vi "main.vi"() -> ()   [LabVIEW 2019]
uses:
  Controls/data.ctl
  Estats.ctl
panel:
  out "Pict Ring":u16(ring)
  in  "Prova":bool
  out "Diners":string
  in  "Stop Button":bool
  out "Diàleg":string
  out "Canvi":string
  in  "Orange":bool
  in  "Lemond":bool
  in  "Apple":bool
  in  "50cents":bool
  in  "20cents":bool
  in  "10cents":bool
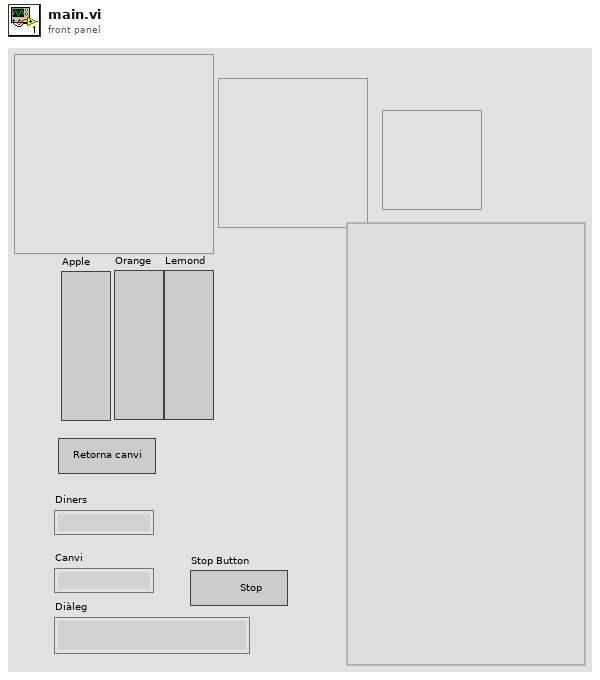
[diagram p1: front panel]
types:
  T1 = typedef "Estats.ctl" = enum16{"Init", "Wait for Event", "Exit", "Return Money", "Lemond", "Apple", "Orange", "Deliver", "50cents", "20cents", "10cents"}
  T2 = typedef "data.ctl" = cluster{"Diners":dbl, "Han triat veguda":bool}
  T3 = enum8{"Enabled", "Disabled", "Disabled and Grayed Out"}
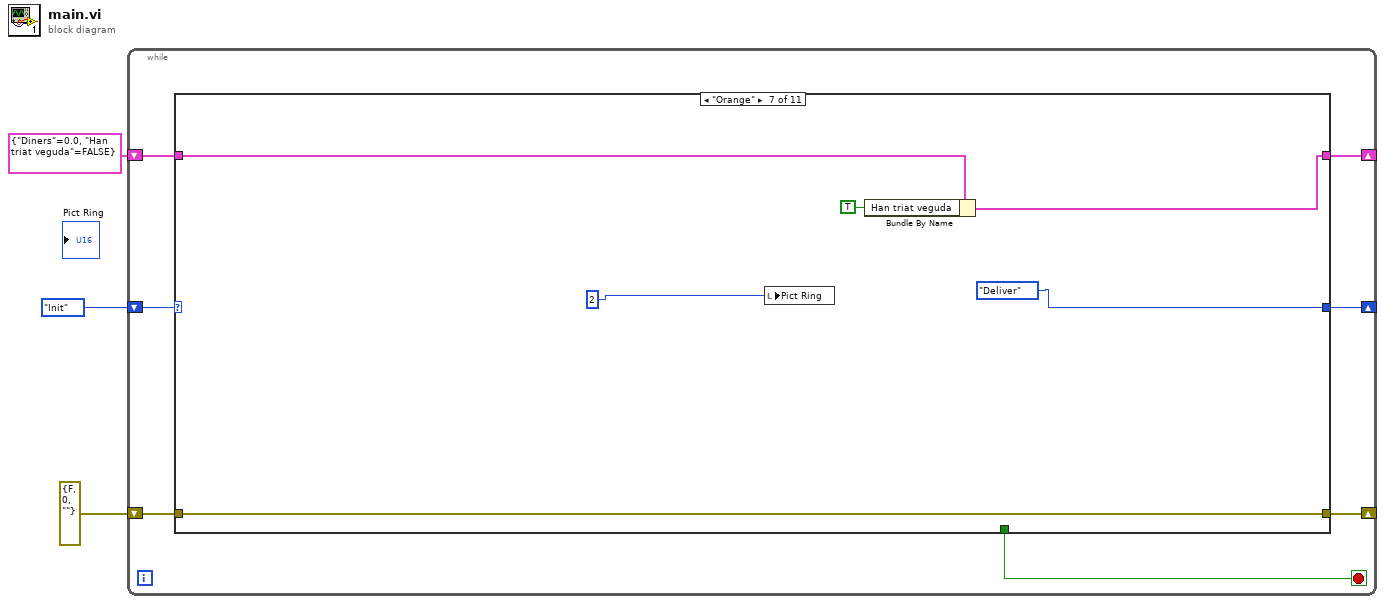
[diagram p0: block diagram]
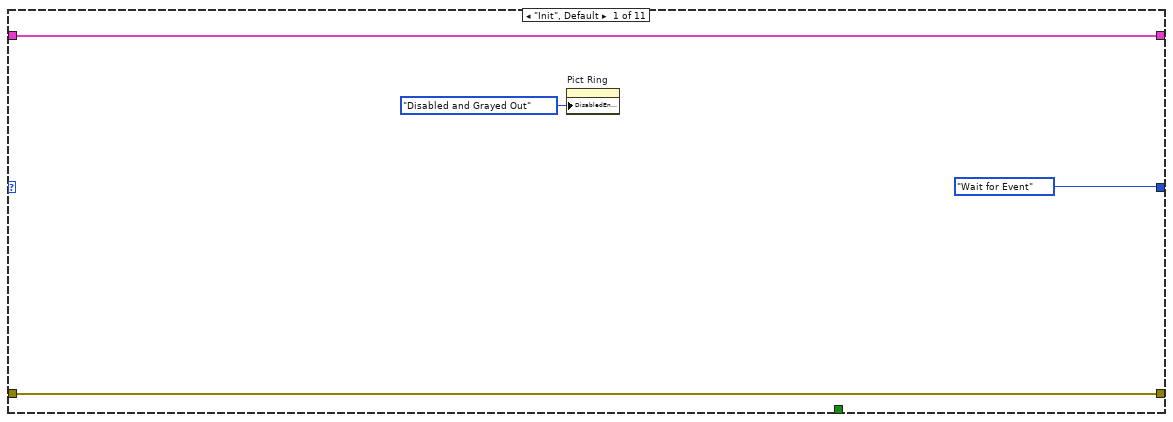
[diagram p2: hidden frame]
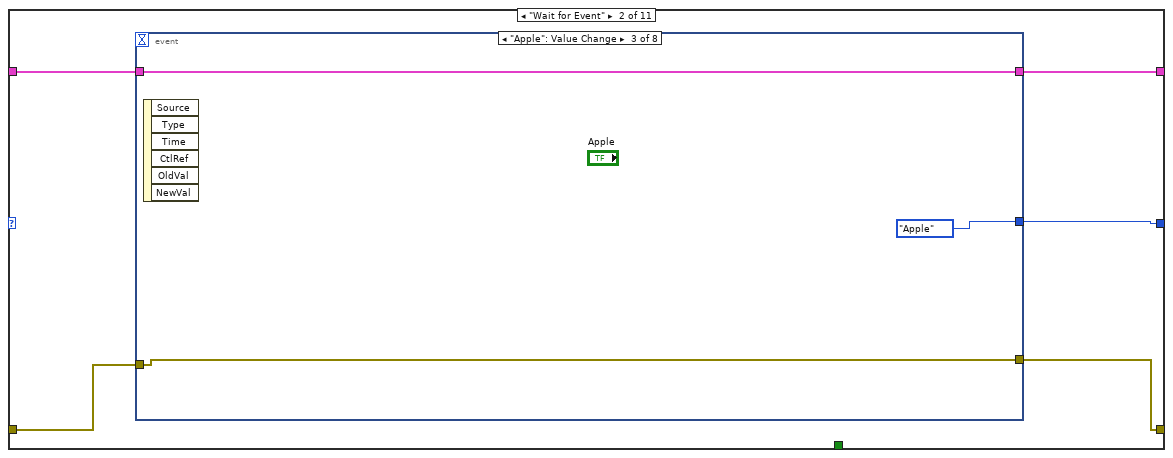
[diagram p3: hidden frame]
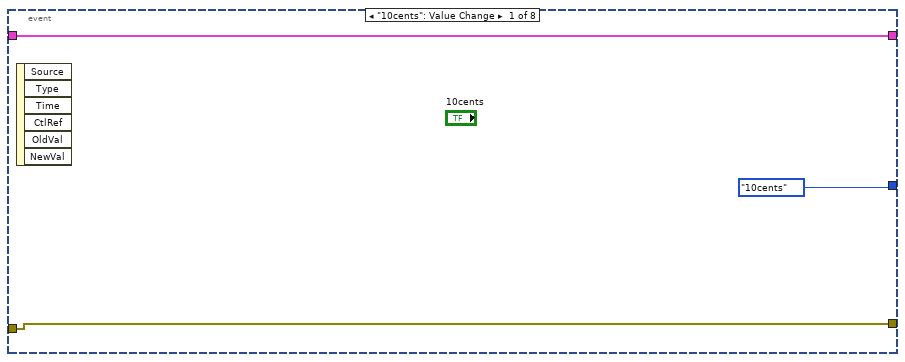
[diagram p4: hidden frame]
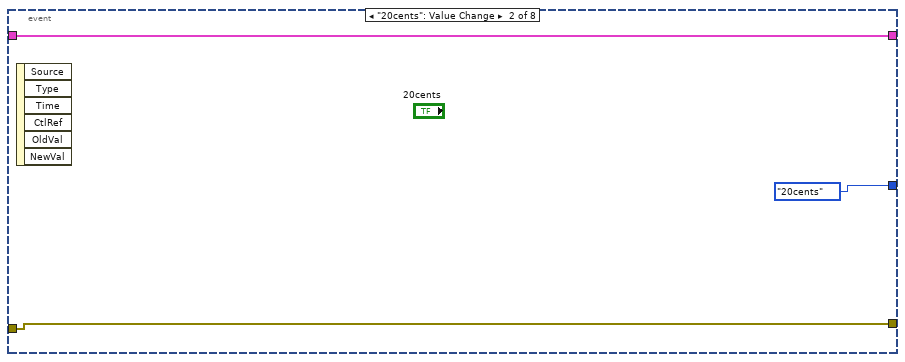
[diagram p5: hidden frame]
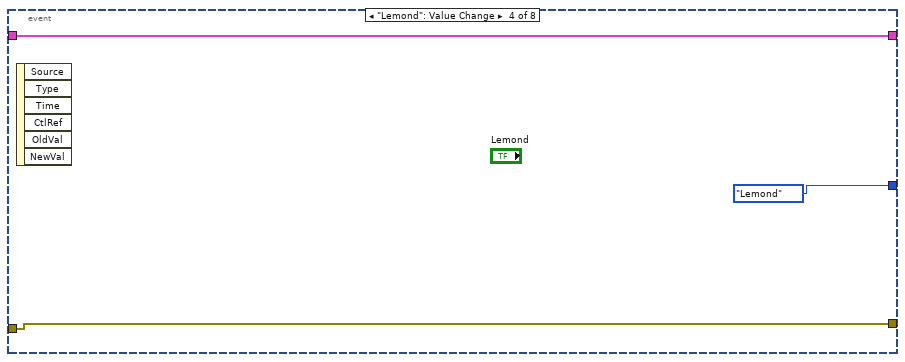
[diagram p6: hidden frame]
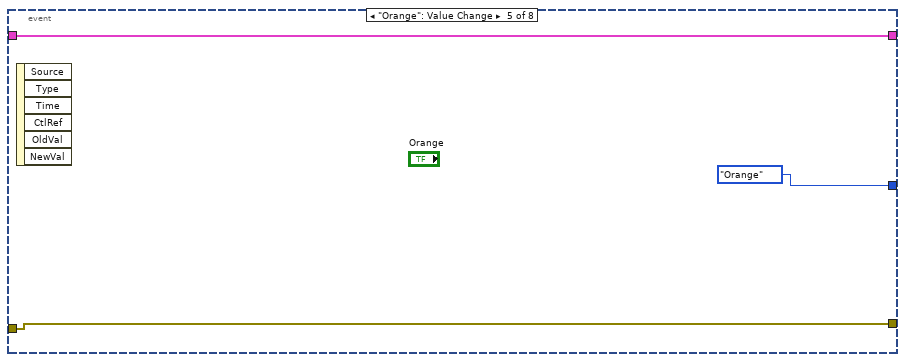
[diagram p7: hidden frame]
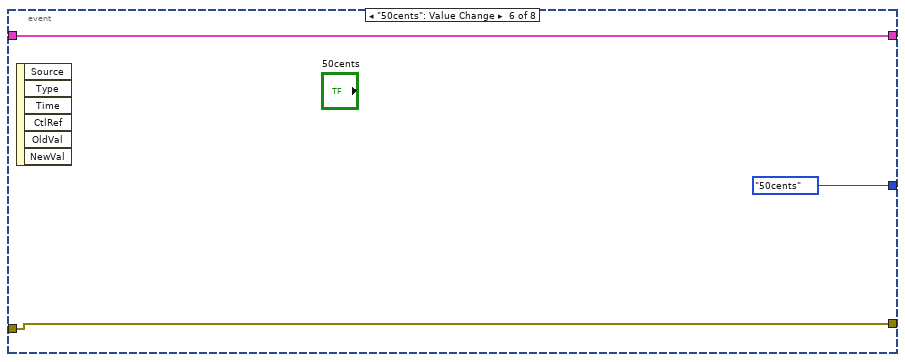
[diagram p8: hidden frame]
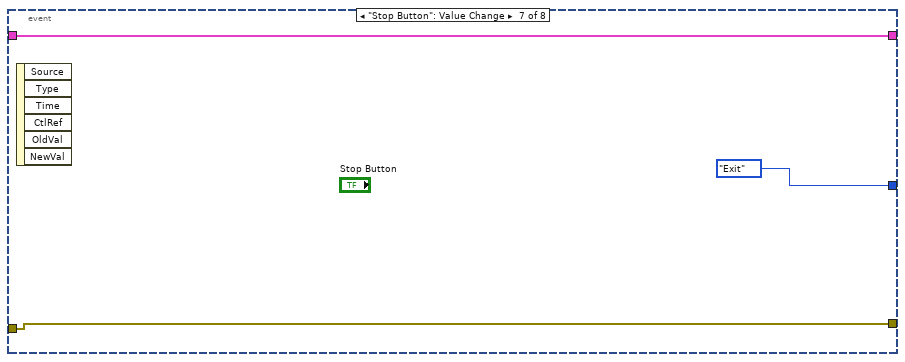
[diagram p9: hidden frame]
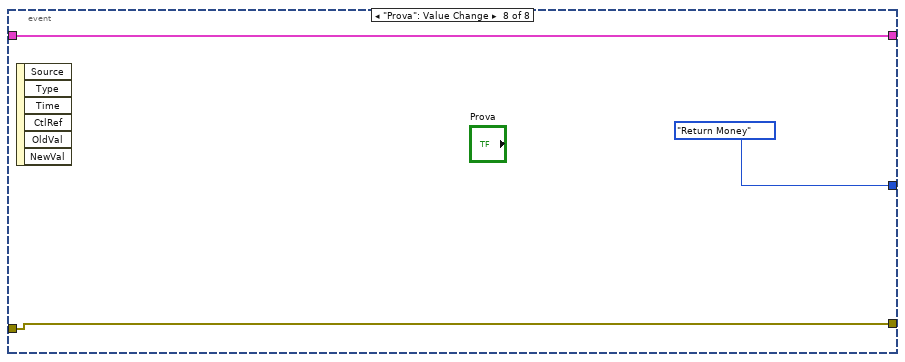
[diagram p10: hidden frame]
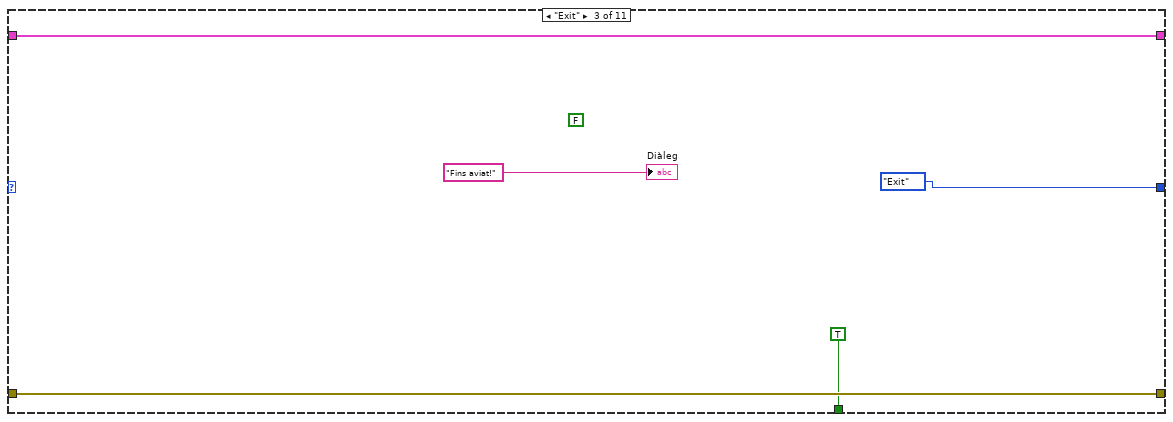
[diagram p11: hidden frame]
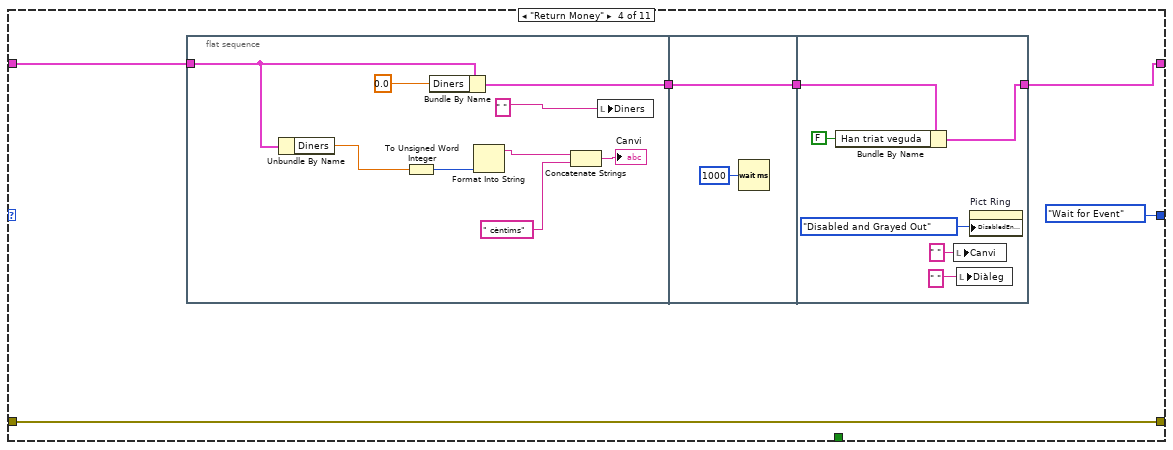
[diagram p12: hidden frame]
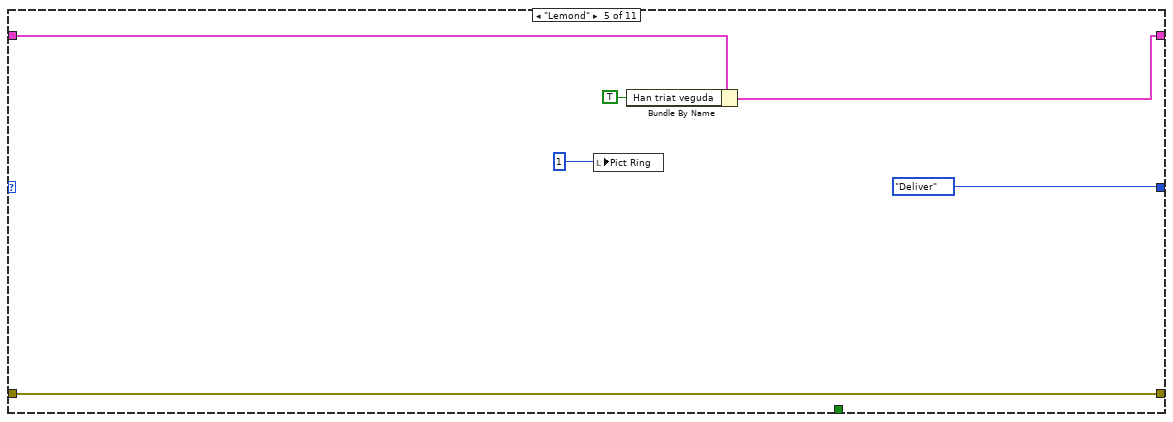
[diagram p13: hidden frame]
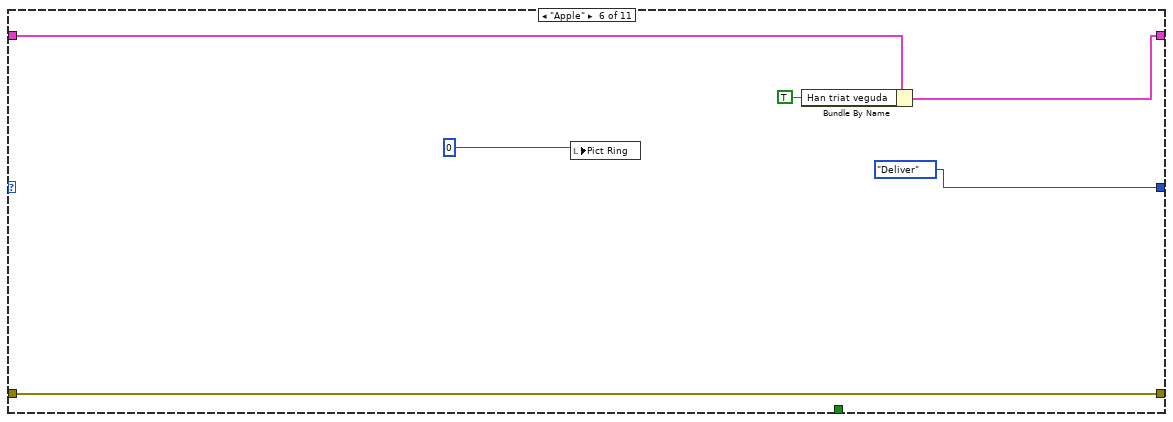
[diagram p14: hidden frame]
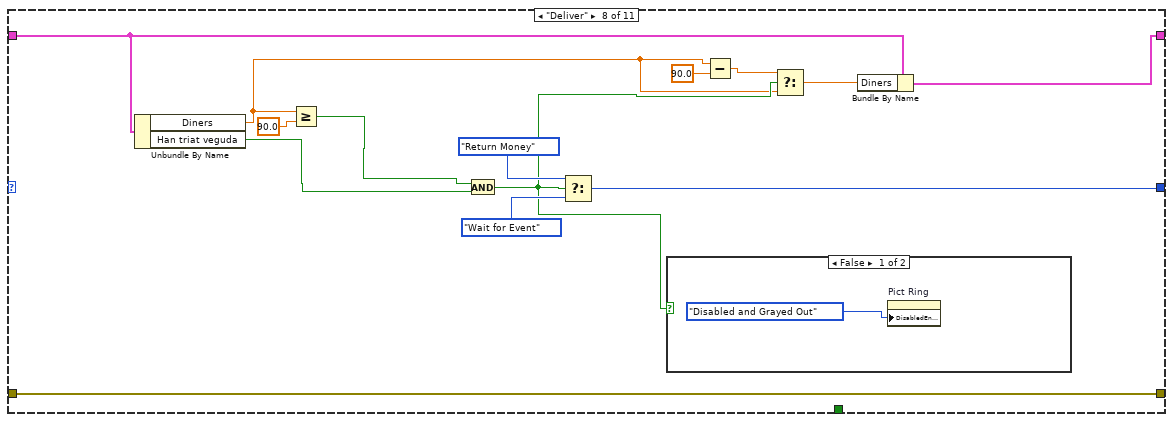
[diagram p15: hidden frame]
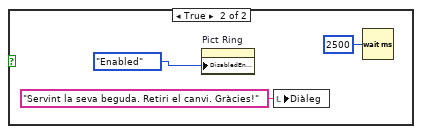
[diagram p16: hidden frame]
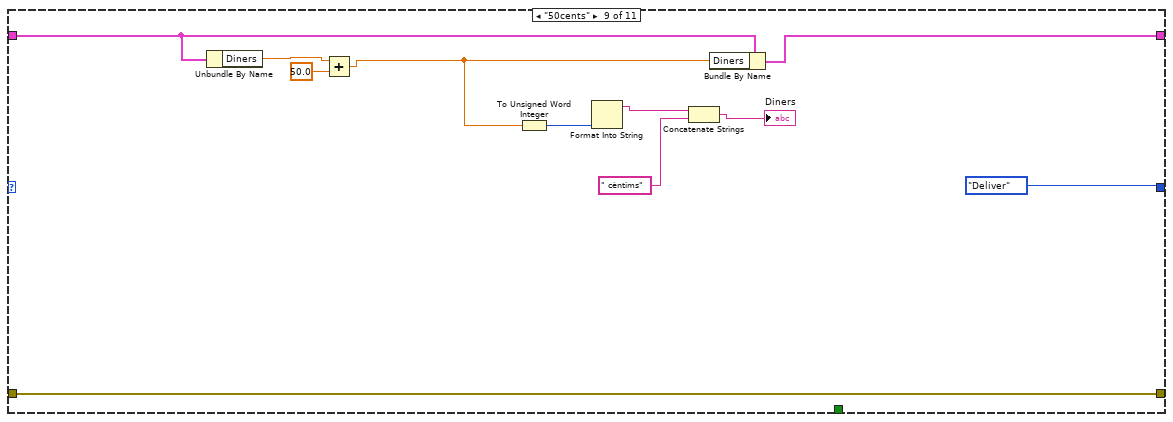
[diagram p17: hidden frame]
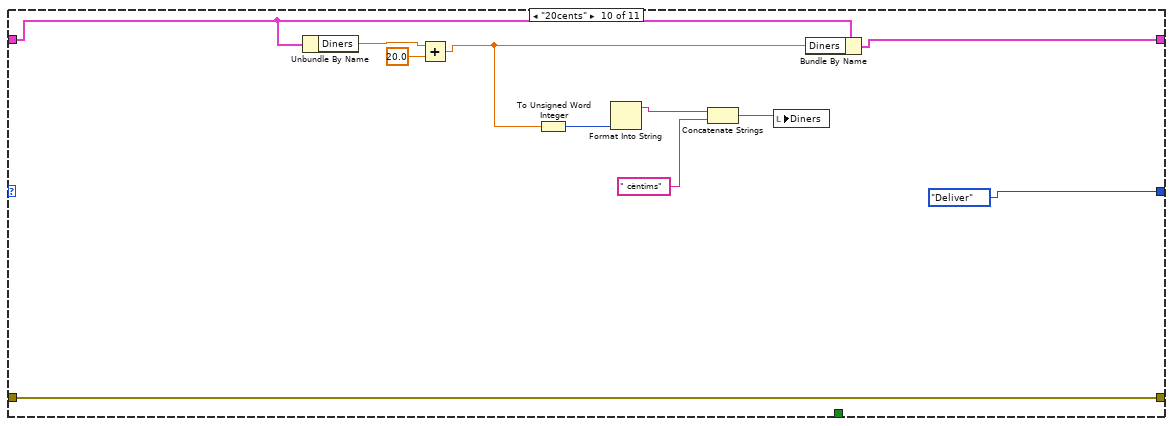
[diagram p18: hidden frame]
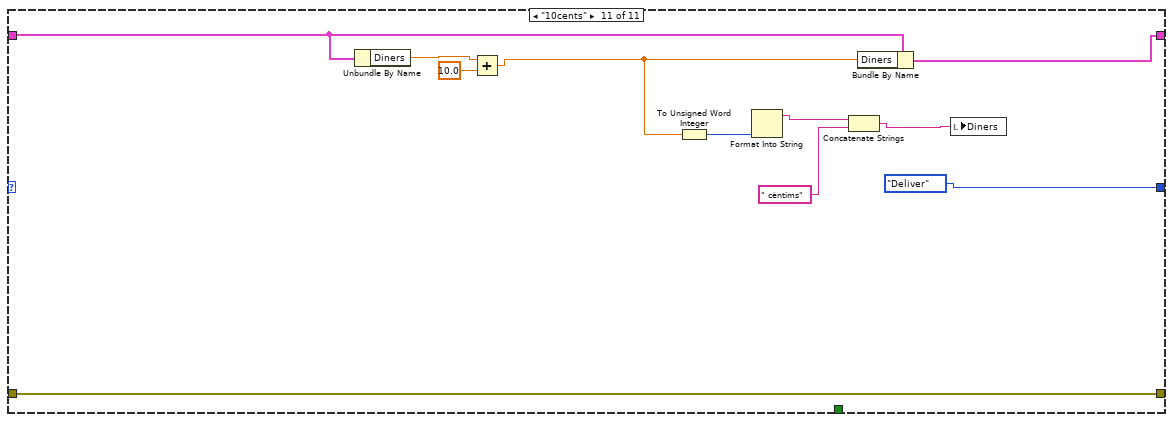
[diagram p19: hidden frame]
diagram:
  n1 = while {
    shift-right: [w5] -> _
    shift-left: Estats."Init" ("Enum") -> [w10]
    shift-right: [w6] -> _
    shift-left: T2 {"Diners"=0.0, "Han triat veguda"=FALSE} ("Cluster") -> [w9]
    shift-right: [w7] -> _
    shift-left: errorcluster {"status"=FALSE, "code"=0, "source"=""} ("error constant") -> [w8]
    stop <- w4 stop-if-true
    n2 = case shown="\"Orange\"" w10 {
      tunnel: w9 -> [w14 w18 w47 w52 w75 w80 w86 w97 w114 w125 w136]
      tunnel: w8 -> [w12 w17 w46 w53 w76 w82 w88 w100 w117 w128 w139]
      tunnel: [w12 w16 w46 w53 w76 w82 w88 w100 w117 w128 w139] -> w7
      tunnel: [w14 w19 w47 w51 w74 w79 w85 w96 w113 w124 w135] -> w6
      tunnel: [Estats."Wait for Event" ("Enum") w15 Estats."Exit" ("Enum") Estats."Wait for Event" ("Enum") Estats."Deliver" ("Enum") Estats."Deliver" ("Enum") Estats."Deliver" ("Enum") w101 Estats."Deliver" ("Enum") Estats."Deliver" ("Enum") Estats."Deliver" ("Enum")] -> w5
      tunnel: [_ _ TRUE ("stop") _ _ _ _ _ _ _ _] -> w4
      frame "Init", Default {
        n3 = property on="Pict Ring" class="Ring (strict)"("DisabledEnum"=T3."Disabled and Grayed Out" ("Disabled")) -> ()  [unwired: 2 in, 2 out]
      }
      frame "Wait for Event" {
        n4 = event shown="[2] \"Apple\": Value Change" {
          selector: _ -> [_ _ _ _ _ _ _ _]
          dyn-events: _ -> [_ _ _ _ _ _ _ _]
          timeout: _ -> [_ _ _ _ _ _ _ _]
          tunnel: [w21 w24 w26 w29 w32 w35 w38 w41] -> w19
          tunnel: w18 -> [w21 w24 w26 w29 w32 w35 w38 w41]
          tunnel: w17 -> [w20 w23 w27 w30 w33 w36 w39 w42]
          tunnel: [w20 w23 w27 w30 w33 w36 w39 w42] -> w16
          tunnel: [Estats."10cents" ("Enum") Estats."20cents" ("Enum") Estats."Apple" ("Enum") Estats."Lemond" ("Enum") Estats."Orange" ("Enum") Estats."50cents" ("Enum") Estats."Exit" ("Enum") Estats."Return Money" ("Enum")] -> w15
          event "10cents": Value Change {
            n5 = event-data() -> ()  [unwired: 1 in, 6 out]
          }
          event "20cents": Value Change {
            n6 = event-data() -> ()  [unwired: 1 in, 6 out]
          }
          event "Apple": Value Change {
            n7 = event-data() -> ()  [unwired: 1 in, 6 out]
          }
          event "Lemond": Value Change {
            n8 = event-data() -> ()  [unwired: 1 in, 6 out]
          }
          event "Orange": Value Change {
            n9 = event-data() -> ()  [unwired: 1 in, 6 out]
          }
          event "50cents": Value Change {
            n10 = event-data() -> ()  [unwired: 1 in, 6 out]
          }
          event "Stop Button": Value Change {
            n11 = event-data() -> ()  [unwired: 1 in, 6 out]
          }
          event "Prova": Value Change {
            n12 = event-data() -> ()  [unwired: 1 in, 6 out]
          }
        }
      }
      frame "Exit" {
        (unwired) FALSE ("Visible")
        "Diàleg" <- "Fins aviat!" ("Estat")
      }
      frame "Return Money" {
        n13 = flat-sequence {
          tunnel: w52 -> [w61]
          tunnel: [w60] -> w50
          tunnel: w50 -> [w65]
          tunnel: [w65] -> w49
          tunnel: [w69] -> w51
          tunnel: w49 -> [w67]
          frame #0 {
            n14 = Unbundle By Name(w61) -> ("Diners"=w58:dbl)
            n15 = To Unsigned Word Integer(number=w58) -> (unsigned 16bit integer=w59:u16)
            n16 = Bundle By Name(cluster=w61, "Diners"=0.0) -> (w60:T2)
            n17 = Format Into String(w59) -> (resulting string=w62:string)  [unwired: 3 in, 1 out]
            n18 = Concatenate Strings(w62, " cèntims" ("string")) -> (→"Canvi":string)
            n19 = local write "Diners"(" " ("Canvi")) -> ()
          }
          frame #1 {
            n20 = Wait (ms)(milliseconds to wait=u32 1000) -> ()  [unwired: 1 out]
          }
          frame #2 {
            n21 = Bundle By Name(cluster=w67, "Han triat veguda"=FALSE) -> (w69:T2)
            n22 = local write "Canvi"(" " ("Canvi")) -> ()
            n23 = local write "Diàleg"(" " ("Canvi")) -> ()
            n24 = property on="Pict Ring" class="Ring (strict)"("DisabledEnum"=T3."Disabled and Grayed Out" ("Disabled")) -> ()  [unwired: 2 in, 2 out]
          }
        }
      }
      frame "Lemond" {
        n25 = local write "Pict Ring"(u16 1 ("Ring")) -> ()
        n26 = Bundle By Name(cluster=w75, "Han triat veguda"=TRUE) -> (w74:T2)
      }
      frame "Apple" {
        n27 = local write "Pict Ring"(u16 0 ("Ring")) -> ()
        n28 = Bundle By Name(cluster=w80, "Han triat veguda"=TRUE) -> (w79:T2)
      }
      frame "Orange" {
        n29 = local write "Pict Ring"(u16 2 ("Ring")) -> ()
        n30 = Bundle By Name(cluster=w86, "Han triat veguda"=TRUE) -> (w85:T2)
      }
      frame "Deliver" {
        n31 = Unbundle By Name(w97) -> ("Diners"=w90:dbl, "Han triat veguda"=w99:bool)
        n32 = Greater Or Equal?(x=w90, y=90.0 ("x")) -> (x >= y?=w98:bool)
        n33 = And(x=w98, y=w99) -> (x .and. y?=w92:bool)
        n34 = Select(t=Estats."Return Money" ("Enum"), s=w92, f=Estats."Wait for Event" ("Enum")) -> (s? t:f=w101:T1)
        n35 = case shown="False" w92 {
          frame False {
            n36 = property on="Pict Ring" class="Ring (strict)"("DisabledEnum"=T3."Disabled and Grayed Out" ("Disabled")) -> ()  [unwired: 2 in, 2 out]
          }
          frame True {
            n37 = property on="Pict Ring" class="Ring (strict)"("DisabledEnum"=T3."Enabled" ("Disabled")) -> ()  [unwired: 2 in, 2 out]
            n38 = local write "Diàleg"("Servint la seva beguda. Retiri el canvi. Gràcies!" ("Estat")) -> ()
            n39 = Wait (ms)(milliseconds to wait=u32 2500) -> ()  [unwired: 1 out]
          }
        }
        n40 = Subtract(x=w90, y=90.0) -> (x-y=w94:dbl)
        n41 = Select(t=w94, s=w92, f=w90) -> (s? t:f=w95:dbl)
        n42 = Bundle By Name(cluster=w97, "Diners"=w95) -> (w96:T2)
      }
      frame "50cents" {
        n43 = Unbundle By Name(w114) -> ("Diners"=w115:dbl)
        n44 = Add(x=w115, y=50.0) -> (x+y=w109:dbl)
        n45 = To Unsigned Word Integer(number=w109) -> (unsigned 16bit integer=w110:u16)
        n46 = Format Into String(w110) -> (resulting string=w108:string)  [unwired: 3 in, 1 out]
        n47 = Concatenate Strings(w108, " cèntims" ("string")) -> (→"Diners":string)
        n48 = Bundle By Name(cluster=w114, "Diners"=w109) -> (w113:T2)
      }
      frame "20cents" {
        n49 = Unbundle By Name(w125) -> ("Diners"=w126:dbl)
        n50 = Add(x=w126, y=20.0) -> (x+y=w120:dbl)
        n51 = To Unsigned Word Integer(number=w120) -> (unsigned 16bit integer=w122:u16)
        n52 = Format Into String(w122) -> (resulting string=w121:string)  [unwired: 3 in, 1 out]
        n53 = Concatenate Strings(w121, " cèntims" ("string")) -> (w119:string)
        n54 = local write "Diners"(w119) -> ()
        n55 = Bundle By Name(cluster=w125, "Diners"=w120) -> (w124:T2)
      }
      frame "10cents" {
        n56 = Unbundle By Name(w136) -> ("Diners"=w137:dbl)
        n57 = Add(x=w137, y=10.0) -> (x+y=w131:dbl)
        n58 = To Unsigned Word Integer(number=w131) -> (unsigned 16bit integer=w133:u16)
        n59 = Format Into String(w133) -> (resulting string=w134:string)  [unwired: 3 in, 1 out]
        n60 = Concatenate Strings(w134, " cèntims" ("string")) -> (w130:string)
        n61 = Bundle By Name(cluster=w136, "Diners"=w131) -> (w135:T2)
        n62 = local write "Diners"(w130) -> ()
      }
    }
  }
